vi "Clear Markers.vi"(7 "Single Marker Address (0)":dbl, 8 "error in (no error)":errorcluster, 9 "Clear Markers (0: Single Marker)":u16(ring) items=["Single Marker", "All Markers"], 10 "Arbitrary Waveform Name":string, 11 "VISA resource name":refnum<visa-resource-name>) -> (0 "error out":errorcluster, 3 "VISA resource name out":refnum<visa-resource-name>)   [LabVIEW 2015, in "Fluke 28x Series.lvlib"]
doc: "Deletes either a single marker, or all markers, from the waveform. \n\n<b>Note</b>: This VI only applies to arbitrary waveforms."
uses:
  <instrlib>/Fluke 28x Series/Fluke 28x Series.lvlib
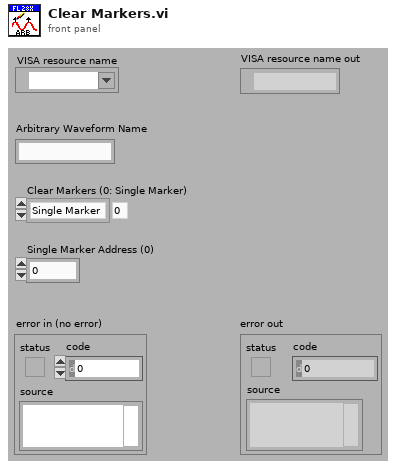
[diagram p1: front panel]
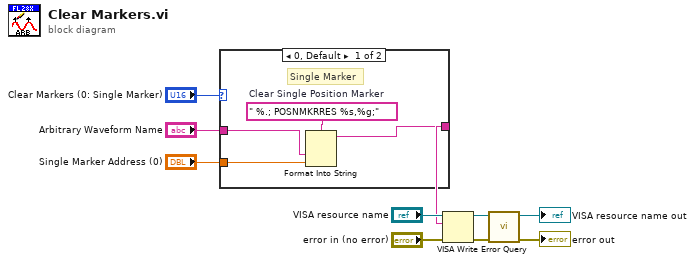
[diagram p0: block diagram]
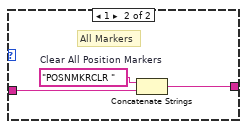
[diagram p2: hidden frame]
diagram:
  n1 = case shown="0, Default" "Clear Markers (0: Single Marker)" {
    tunnel: "Single Marker Address (0)" -> [w13 _]
    tunnel: "Arbitrary Waveform Name" -> [w12 w16]
    tunnel: [w11 w15] -> w2
    frame 0, Default {
      w14 = " %.; POSNMKRRES %s,%g;"  # Clear Single Position Marker
      # "Single Marker"
      n2 = Format Into String(format string=w14, w12, w13) -> (resulting string=w11:string)  [unwired: 2 in, 1 out]
    }
    frame 1 {
      w17 = "POSNMKRCLR "  # Clear All Position Markers
      # "All Markers"
      n3 = Concatenate Strings(w17, w16) -> (w15:string)
    }
  }
  n4 = VISA Write(VISA resource name="VISA resource name", write buffer=w2, error in (no error)="error in (no error)") -> (VISA resource name out=w9:refnum<visa-resource-name>, error out=w8:errorcluster)  [unwired: 1 out]
  n5 = call <instrlib>:"Error Query.vi"("error in (no error)"=w8, "VISA resource name"=w9) -> ("error out"=→"error out":errorcluster, "VISA resource name out"=→"VISA resource name out":refnum<visa-resource-name>)  [unwired: 6 in, 2 out]
